vi "UMLEditor UpdateMethodsAttributesDialog.vi"(1 "OldAttributesIn":string, 2 "OldMethodsIn":string, 3 "New Attributes":string, 4 "New Methods":string, 5 "error in (no error)":errorcluster) -> (15 "AttributesOut":string, 16 "MethodsOut":string, 18 "CancelOut":bool, 19 "error out":errorcluster)   [LabVIEW 2012]
panel:
  in  "Cancel":bool
  in  "OK":bool
  out "Old Methods":string
  out "Old Attributes":string
  # "This shows the new attributes and methods, \nthat will be used.\nYou can update now before applying changes"
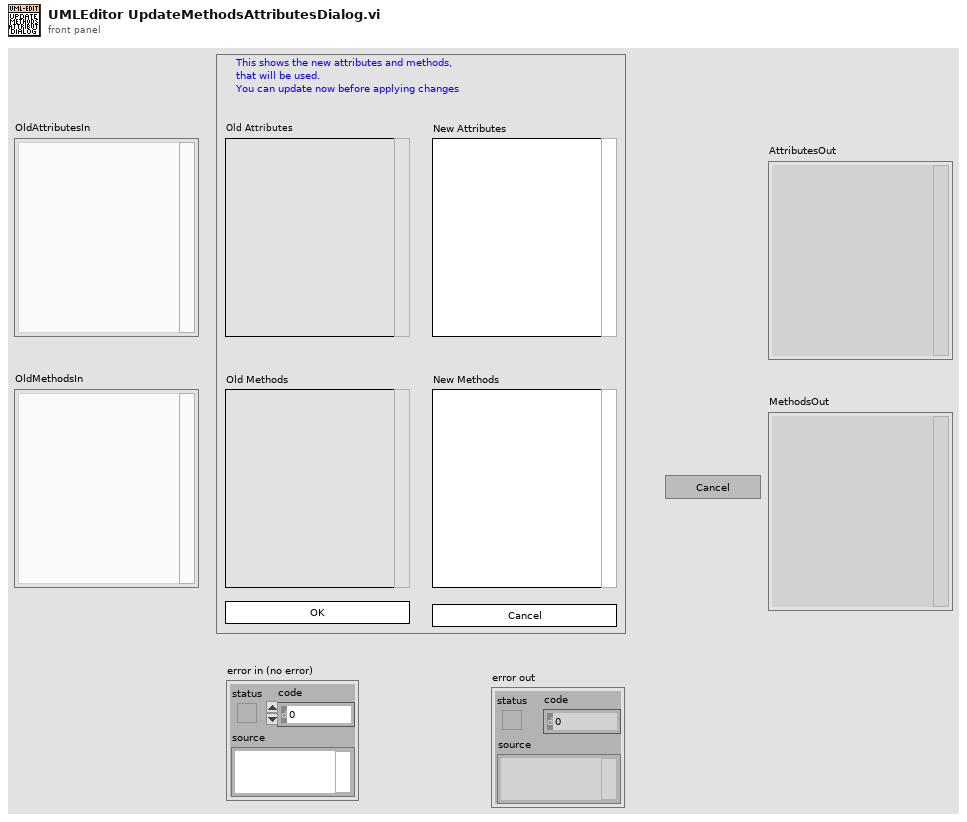
[diagram p1: front panel]
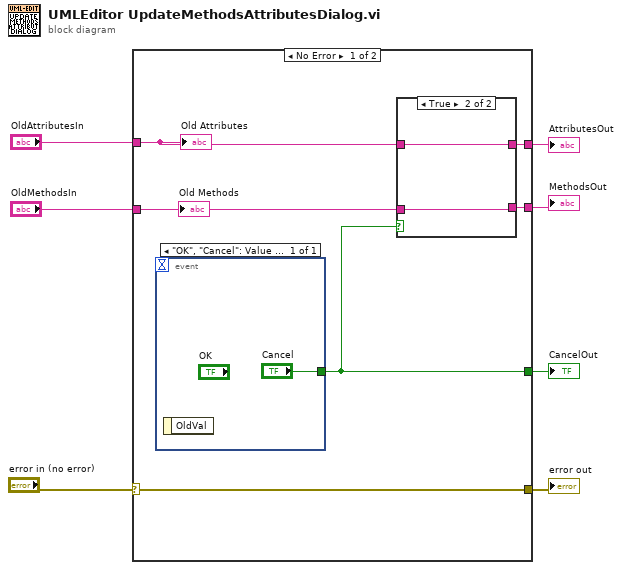
[diagram p0: block diagram]
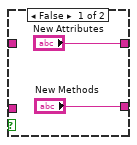
[diagram p2: hidden frame]
diagram:
  n1 = case shown="No Error" "error in (no error)" {
    selector: "error in (no error)" -> [w8 w19]
    tunnel: [w13 _] -> w7
    tunnel: [w12 _] -> w6
    tunnel: [w11 _] -> w5
    tunnel: "OldAttributesIn" -> [w10 _]
    tunnel: "OldMethodsIn" -> [w9 _]
    tunnel: [w8 w19] -> w1
    frame No Error {
      n2 = event shown="[0] \"OK\", \"Cancel\": Value Change" {
        selector: _ -> [_]
        dyn-events: _ -> [_]
        timeout: _ -> [_]
        tunnel: ["Cancel"] -> w13
        event "OK", "Cancel": Value Change {
          n3 = event-data() -> ()  [unwired: 2 out]
        }
      }
      n4 = case shown="True" w13 {
        tunnel: ["New Attributes" w17] -> w12
        tunnel: ["New Methods" w16] -> w11
        tunnel: w10 -> [_ w17]
        tunnel: w9 -> [_ w16]
        frame False {
        }
        frame True {
        }
      }
      "Old Attributes" <- w10
      "Old Methods" <- w9
    }
    frame Error {
    }
  }
  "CancelOut" <- w7
  "AttributesOut" <- w6
  "MethodsOut" <- w5
  "error out" <- w1
